vi "set_movie_start_time.vi"(8 "error in (no error)":errorcluster, 10 "movie start":timestamp, 11 "ImageCollection.lvclass in":refnum<class "ImageCollection.lvclass">) -> (0 "error out":errorcluster, 3 "ImageCollection.lvclass out":refnum<class "ImageCollection.lvclass">)   [LabVIEW 2010, in "ImageCollection.lvclass"]
uses:
  ImageCollection.lvclass
  ImageCollection.lvclass/ImageCollection.ctl
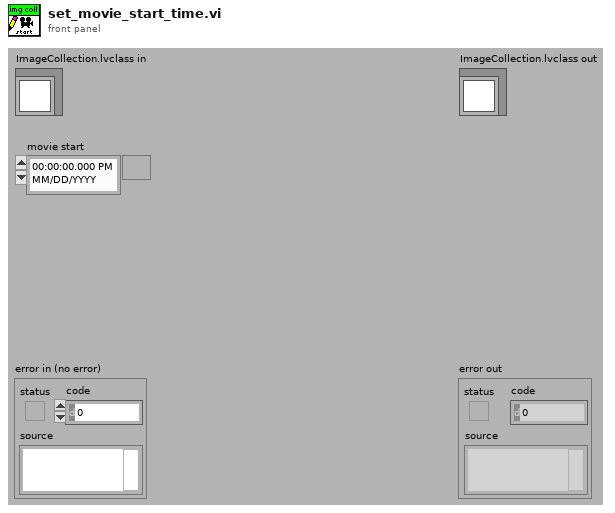
[diagram p1: front panel]
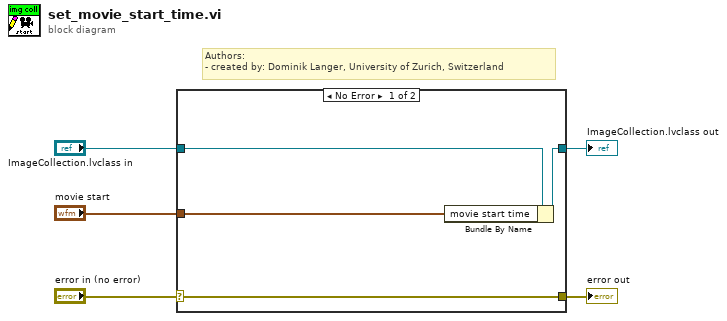
[diagram p0: block diagram]
diagram:
  # "Authors: \n- created by: Dominik Langer, University of Zurich, Switzerland"
  n1 = case shown="No Error" "error in (no error)" {
    selector: "error in (no error)" -> [w9 w10]
    tunnel: [w9 w10] -> w4
    tunnel: [w7 w11] -> w2
    tunnel: "ImageCollection.lvclass in" -> [w8 w11]
    tunnel: "movie start" -> [w6 _]
    frame No Error {
      n2 = Bundle By Name(cluster=w8, "movie start time"=w6) -> (w7:refnum<class "ImageCollection.lvclass">)
    }
    frame Error {
    }
  }
  "error out" <- w4
  "ImageCollection.lvclass out" <- w2
